vi "Config Measure User Define.vi"(0 "VISA resource name":refnum<visa-resource-name>, 1 "Function No (1: Function 1)":u16(ring)=1 items=["", "Function 1", "Function 2", "Function 3", "Function 4"], 5 "State (F: OFF)":bool, 11 "error in (no error)":errorcluster, 12 "Expression ( URMS(E1) )":string="URMS(E1)", 13 "Unit (V)":string="V") -> (4 "VISA resource name out":refnum<visa-resource-name>, 15 "error out":errorcluster)   [LabVIEW 2013, in "Yokogawa PZ4000.lvlib"]
doc: "This VI sends the Measure User Define group command to the PZ4000 series."
uses:
  Yokogawa PZ4000.lvlib
panel:
  # "ON\nOFF"
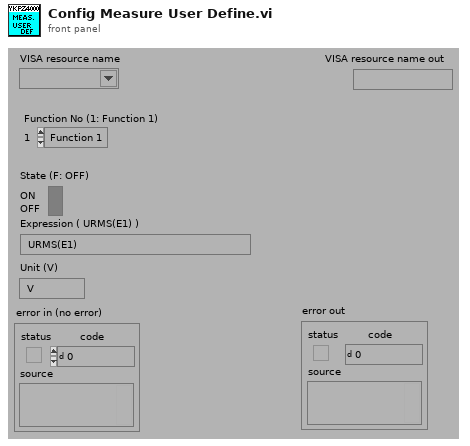
[diagram p1: front panel]
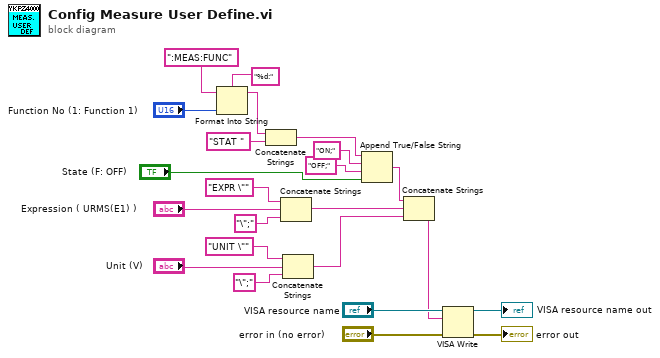
[diagram p0: block diagram]
diagram:
  n1 = Format Into String(format string="%d:", initial string=":MEAS:FUNC", "Function No (1: Function 1)") -> (resulting string=w12:string)  [unwired: 1 in, 1 out]
  n2 = Concatenate Strings(w12, "STAT ") -> (w13:string)
  n3 = Concatenate Strings("EXPR \"", "Expression ( URMS(E1) )", "\";") -> (w3:string)
  n4 = Concatenate Strings("UNIT \"", "Unit (V)", "\";") -> (w2:string)
  n5 = Append True/False String(1:"State (F: OFF)", 2:"OFF;", 3:"ON;", 4:w13) -> (0:w5:string)
  n6 = Concatenate Strings(w5, w3, w2) -> (w4:string)
  n7 = VISA Write(VISA resource name="VISA resource name", write buffer=w4, error in (no error)="error in (no error)") -> (VISA resource name out=→"VISA resource name out":refnum<visa-resource-name>, error out=→"error out":errorcluster)  [unwired: 1 out]
